vi "Remove 1frame tracks.vi"(10 "count array in":i32[](array[numeric])) -> (2 "count array out":i32[](array[numeric]))   [LabVIEW 2014]
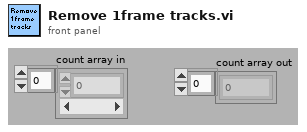
[diagram p1: front panel]
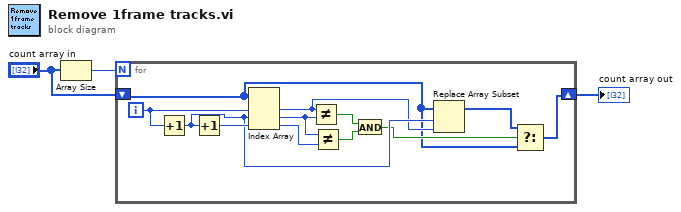
[diagram p0: block diagram]
diagram:
  n1 = Array Size(array="count array in") -> (size(s)=w3:i32)
  n2 = for {
    N: w3 -> [_]
    shift-right: [w4] -> w1
    shift-left: "count array in" -> [w5]
    i -> [w15]
    n3 = Increment(x=w15) -> (x+1=w9:i32)
    n4 = Increment(x=w9) -> (x+1=w14:i32)
    n5 = Index Array(array=w5, index #1=w15, index #2=w9, index #3=w14) -> (element #1=w8:i32, element #2=w10:i32, element #3=w13:i32)
    n6 = Not Equal?(x=w8, y=w10) -> (x != y?=w12:bool)
    n7 = Not Equal?(x=w10, y=w13) -> (x != y?=w11:bool)
    n8 = And(x=w12, y=w11) -> (x .and. y?=w7:bool)
    n9 = Replace Array Subset(array=w5, new element=w8, index=w9) -> (w6:i32[])
    n10 = Select(t=w6, s=w7, f=w5) -> (s? t:f=w4:i32[])
  }
  "count array out" <- w1
